vi "optionsAcq_PDTemperatureMode.vi"(0 "reference":refnum<class "OSA200.lvclass">, 2 "PD sensitivity mode":T1, 5 "error in (no error)":errorcluster, 9 "read/write":enum16{"read", "write"}(ring)) -> (14 "duplicate reference":refnum<class "OSA200.lvclass">, 16 "PD sensitivity mode out":T1, 18 "PD senseMode implemented":bool, 19 "error out":errorcluster)   [LabVIEW 2010, in "OSA200.lvclass"]
doc: "The OSA optical detectors in some models are cooled to improve the noise floor, (typically cooled at -30 degrees C for a reduction of thermal noise). However the cooling also restricts the upper wavelength range which is why a warm detector temperature mode can be selected to extend the range.\n[OSA200]"
uses:
  OSA200.lvclass
  _misc/Thorlabs_FTS_misc.llb/PDTemperatureMode.ctl
  OSA.lvclass
  OSA20X_misc.lvlib
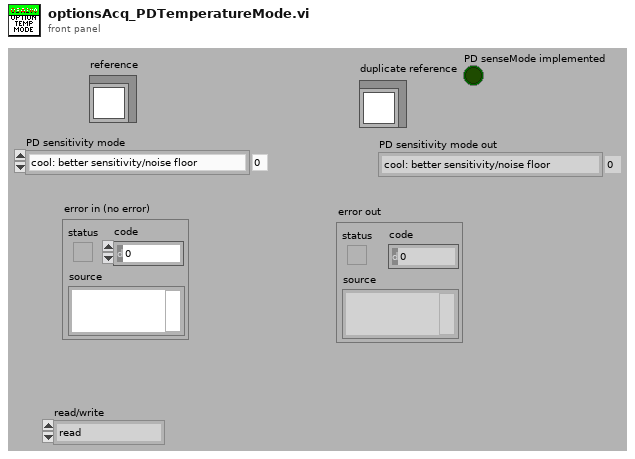
[diagram p1: front panel]
types:
  T1 = typedef "OSA20X_misc.lvlib/PDTemperatureMode.ctl" = enum16{"cool: better sensitivity/noise floor", "warm: extended wl range"}
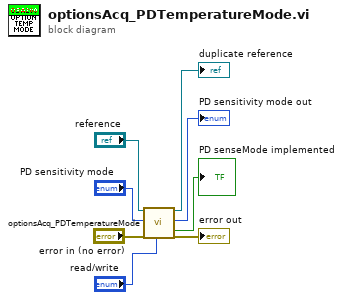
[diagram p0: block diagram]
diagram:
  n1 = call-parent "optionsAcq_PDTemperatureMode.vi"("reference"="reference", "PD sensitivity mode"="PD sensitivity mode", "error in (no error)"="error in (no error)", "read/write"="read/write") -> ("duplicate reference"=→"duplicate reference":refnum<class "OSA200.lvclass">, "PD sensitivity mode out"=→"PD sensitivity mode out":T1, "PD senseMode implemented"=→"PD senseMode implemented":bool, "error out"=→"error out":errorcluster)  [unwired: 12 in]
